vi "Coord window-PictureMap set tip strip.vi"   [LabVIEW 2020]
uses:
  Globals/Coord window-Globals.vi
types:
  T1 = typedef "Coordinate list window refs.ctl" = cluster{"Window Name (i.e. Key)":string, "menu reference":refnum<k9>, "VI's reference":refnum<vi>, "Pane 1":refnum<vi>, "Pane 2":refnum<vi>, "Coord Listbox":refnum<vi>, "File name":refnum<vi>, "Picture Map":refnum<vi>, "Stage XYZ Position ind.":refnum<vi>}
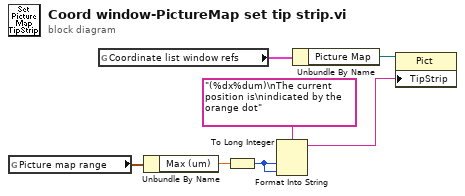
[diagram p0: block diagram]
diagram:
  n1 = global read "Coord window-Globals.vi" "Picture map range"() -> (w5:cluster{"Min (um)":dbl, "Max (um)":dbl})
  n2 = global read "Coord window-Globals.vi" "Coordinate list window refs"() -> (w7:T1)
  n3 = Unbundle By Name(w5) -> ("Max (um)"=w3:dbl)
  n4 = To Long Integer(number=w3) -> (32bit integer=w1:i32)
  n5 = Format Into String(format string="(%dx%dum)\nThe current position is\nindicated by the orange dot", w1, w1) -> (resulting string=w2:string)  [unwired: 2 in, 1 out]
  n6 = Unbundle By Name(w7) -> ("Picture Map"=w6:refnum<vi>)
  n7 = property class="Pict"(reference=w6, "TipStrip"=w2) -> ()  [unwired: 1 in, 2 out]
